vi "InterfaceClientLV.vi"() -> ()   [LabVIEW 2021]
doc: "Le protocole UDP diffère du protocole TCP car il n'y a pas de détection d'erreur avec les paquets d'informations qui sont envoyés ; il n'y a donc aucune garantie qu'un destinataire reçoive bien des données.\n\nLe protocole UDP offre la possibilité de diffuser des données sur un réseau. Spécifiez simplement une adresse IP de uns (255.255.255.255) pour essayer de diffuser l'information sur tout le réseau. Gardez à l'esprit que des routeurs et d'autres périphériques de réseau refusent généralement de diffuser au-delà de certains points, la diffusion est donc limitée dans la pratique."
panel:
  out "chaîne":string
  out "Erreur UDP WRITE":string=" INSTRUCTIONS :\r\rUtilisation normale : Quand vous utilisez des sous-VIs qui incluent la structure entrée/sortie d'erreur, placez ce gestionnaire d'erreur à l'endroit où vous voulez informer l'utilisateur sur une éventuelle erreur, typiquement à la fin d'un bloc d'acquisition de données, comme dernière action du programme.  Si le booléen d'entrée d'erreur affiche ERREUR, le gestionnaire crée un message de description et de la source de l'erreur.  Si le type de dialogue est 1 (valeur par défaut), le message est affiché dans une boîte de dialogue que l'utilisateur doit valider.  Si le type est 2, l'utilisateur peut accuser réception du message ou interrompre l'exécution ; il n'est pas conseillé d'abandonner un programme en train d'effectuer une acquisition.  Si le type est 0, aucun message n'est affiché ; ceci est utilisé pour traiter les erreurs par programmation, et les éléments du cluster de sortie d'erreur sont câblés pour cette raison à des terminaux individuels.  \r\rAutre utilisation :\n\r\nTest local.  Pour tester le code d'erreur d'un sous-VI ou d'une fonction n'ayant pas la structure d'E/S d'erreurs, vous pouvez câbler son code d'erreur et sa chaîne source aux entrées locales code d'erreur et source d'erreur.  Si le booléen d'entrée d'erreur affiche pas d'erreur et si code d'erreur n'est pas nul, le code et la source locale sont substitués aux valeurs d'entrée d'erreur et erreur? passe à VRAI (ERREUR)." caption="message"
  out "sortie d'erreur":errorcluster
  out "Erreur UDP":string=" INSTRUCTIONS :\r\rUtilisation normale : Quand vous utilisez des sous-VIs qui incluent la structure entrée/sortie d'erreur, placez ce gestionnaire d'erreur à l'endroit où vous voulez informer l'utilisateur sur une éventuelle erreur, typiquement à la fin d'un bloc d'acquisition de données, comme dernière action du programme.  Si le booléen d'entrée d'erreur affiche ERREUR, le gestionnaire crée un message de description et de la source de l'erreur.  Si le type de dialogue est 1 (valeur par défaut), le message est affiché dans une boîte de dialogue que l'utilisateur doit valider.  Si le type est 2, l'utilisateur peut accuser réception du message ou interrompre l'exécution ; il n'est pas conseillé d'abandonner un programme en train d'effectuer une acquisition.  Si le type est 0, aucun message n'est affiché ; ceci est utilisé pour traiter les erreurs par programmation, et les éléments du cluster de sortie d'erreur sont câblés pour cette raison à des terminaux individuels.  \r\rAutre utilisation :\n\r\nTest local.  Pour tester le code d'erreur d'un sous-VI ou d'une fonction n'ayant pas la structure d'E/S d'erreurs, vous pouvez câbler son code d'erreur et sa chaîne source aux entrées locales code d'erreur et source d'erreur.  Si le booléen d'entrée d'erreur affiche pas d'erreur et si code d'erreur n'est pas nul, le code et la source locale sont substitués aux valeurs d'entrée d'erreur et erreur? passe à VRAI (ERREUR)." caption="message"
  in  "Période (en ms)":u32=1000 min=500 max=10000 step=500
  out "(sup.inf)":u16
  out "entier 16 bits non signé":u16[](array[numeric])
  out "*(type *) &x":string
  out "sous-tableau":u8[](array[numeric])
  out "Graphe déroulant":dbl(graph)
  out "Cmd [ V | F | A0 | A1 ] 2":i8[](array[numeric])
  in  "Instruction\n[1] Get Analog\n[2] Set Digital (PWM)":u8=1 min=1 max=2
  out "Réponse":u8[](array[numeric])
  in  "Arrêter":bool
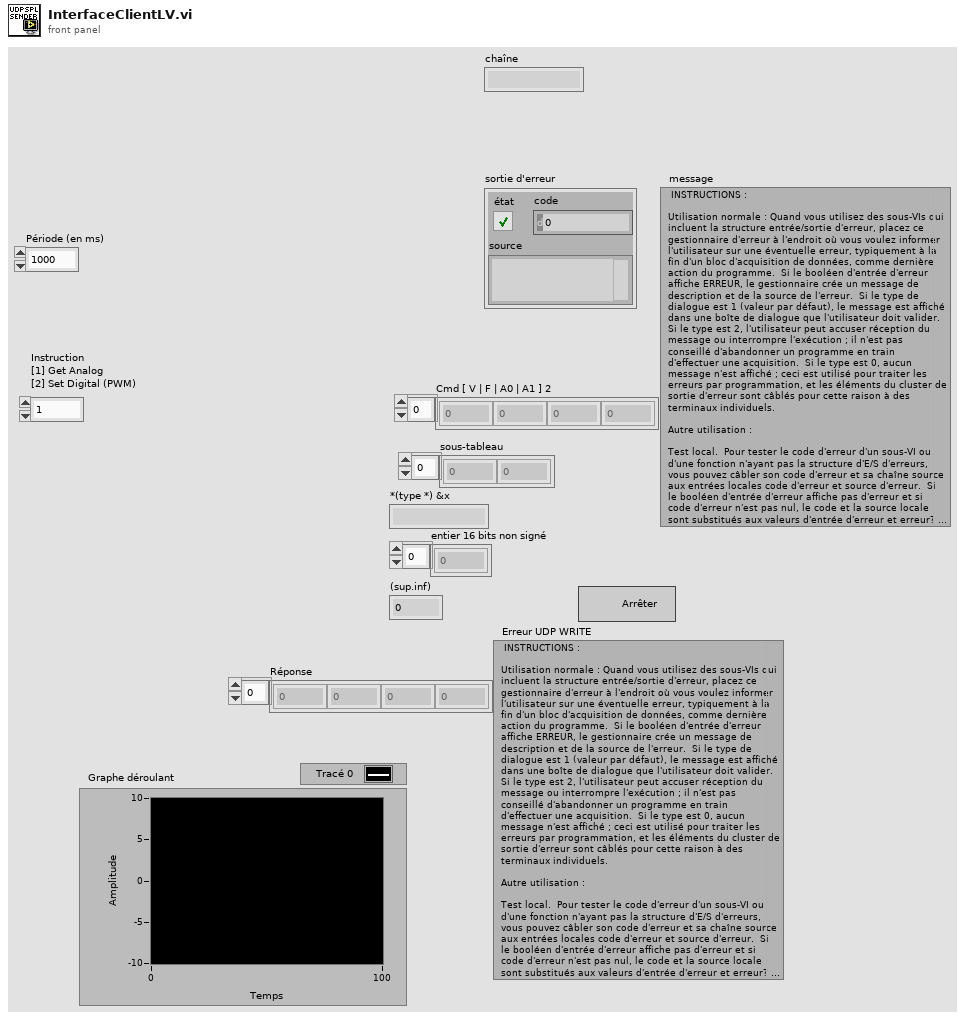
[diagram p1: front panel]
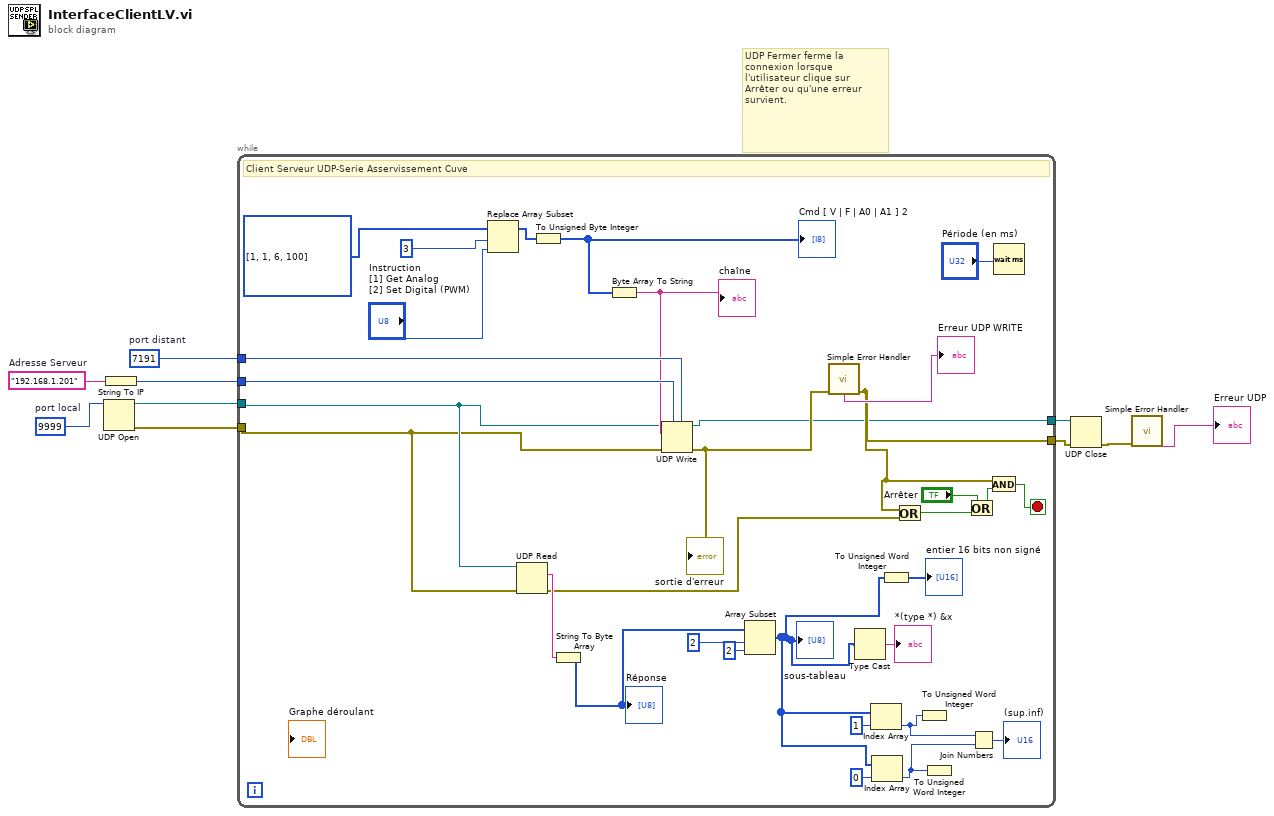
[diagram p0: block diagram]
diagram:
  w5 = u16 7191  # port distant
  w6 = u16 9999  # port local
  w10 = "192.168.1.201"  # Adresse Serveur
  # "UDP Fermer ferme la connexion lorsque l'utilisateur clique sur Arrêter ou qu'une erreur survient."
  n1 = UDP Open(11:w6) -> (port=w8:refnum<k16>, 0:w7:errorcluster)  [unwired: 4 in, 1 out]
  n2 = String To IP(1:w10) -> (0:w9:u32)
  n3 = while {
    tunnel: w8 -> [w39]
    tunnel: w7 -> [w26]
    tunnel: w9 -> [w42]
    tunnel: w5 -> [w41]
    tunnel: [w12] -> w3
    tunnel: [w11] -> w2
    stop <- w20 stop-if-true
    # "Client Serveur UDP-Serie Asservissement Cuve"
    n4 = Replace Array Subset(array=i32[] [1, 1, 6, 100], new element="Instruction\n[1] Get Analog\n[2] Set Digital (PWM)", index=3 ("indice")) -> (w13:i32[])
    n5 = UDP Read(connection ID=w39, 8:w26) -> (data out=w38:string, error out=w25:errorcluster)  [unwired: 2 in, 3 out]
    n6 = To Unsigned Byte Integer(number=w13) -> (unsigned 8bit integer=w21:u8[])
    "Cmd [ V | F | A0 | A1 ] 2" <- w21
    n7 = String To Byte Array(string=w38) -> (unsigned byte array=w37:u8[])
    "Réponse" <- w37
    n8 = Byte Array To String(unsigned byte array=w21) -> (string=w40:string)
    "chaîne" <- w40
    n9 = UDP Write(address=w42, port or service name=w41, connection ID=w39, data in=w40, 8:w26) -> (error out=w18:errorcluster, 3:w11:refnum<k16>)  [unwired: 1 in]
    "sortie d'erreur" <- w18
    n10 = Array Subset(array=w37, index=2 ("indice"), length=2 ("longueur")) -> (w30:u8[])
    "sous-tableau" <- w30
    n11 = call <vilib>:"Simple Error Handler.vi"("error in (no error)"=w18) -> ("error out"=w12:errorcluster, "message"=→"Erreur UDP WRITE":string)  [unwired: 4 in, 3 out]
    n12 = Type Cast(x=w30) -> (*(type *) &x=→"*(type *) &x":string)  [unwired: 1 in]
    n13 = Index Array(array=w30, index=1 ("indice")) -> (element=w29:u8)
    n14 = Index Array(array=w30, index=0 ("indice")) -> (element=w28:u8)
    n15 = To Unsigned Word Integer(number=w30) -> (unsigned 16bit integer=→"entier 16 bits non signé":u16[])
    n16 = Or(x=w12, y=w25) -> (x .or. y?=w24:bool)
    n17 = To Unsigned Word Integer(number=w29) -> ()  [unwired: 1 out]
    n18 = To Unsigned Word Integer(number=w28) -> ()  [unwired: 1 out]
    n19 = Or(x="Arrêter", y=w24) -> (x .or. y?=w19:bool)
    n20 = Join Numbers(hi=w29, lo=w28) -> ((hi.lo)=→"(sup.inf)":u16)
    n21 = And(x=w12, y=w19) -> (x .and. y?=w20:bool)
    n22 = Wait (ms)(milliseconds to wait="Période (en ms)") -> ()  [unwired: 1 out]
  }
  n23 = UDP Close(connection ID=w2, 8:w3) -> (error out=w1:errorcluster)  [unwired: 1 out]
  n24 = call <vilib>:"Simple Error Handler.vi"("error in (no error)"=w1) -> ("message"=→"Erreur UDP":string)  [unwired: 4 in, 4 out]
